vi "电阻有效性判断.vi"(6 "温度值":dbl, 9 "Column":i32=-2, 10 "行数":i32, 11 "Table输入":refnum<vi>) -> ()   [LabVIEW 2015]
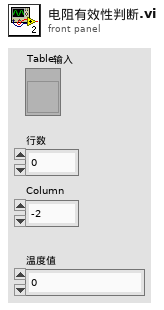
[diagram p1: front panel]
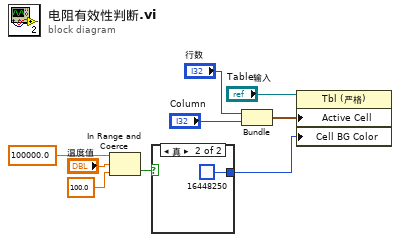
[diagram p0: block diagram]
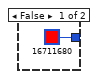
[diagram p2: hidden frame]
diagram:
  n1 = In Range and Coerce(upper limit=100000.0, x="温度值", lower limit=100.0) -> (In Range?=w3:bool)  [unwired: 1 out]
  n2 = case shown="真" w3 {
    tunnel: [u32 16711680 ("Origin BK Color") u32 16448250 ("Origin BK Color")] -> w9
    frame False {
    }
    frame True {
    }
  }
  n3 = Bundle("行数"="行数", "Column"="Column") -> (w8:cluster{"行数":i32, "Column":i32})  [unwired: 1 in]
  n4 = property class="Tbl (严格)"(reference="Table输入", "Active Cell"=w8, "Cell BG Color"=w9) -> ()  [unwired: 1 in, 2 out]
